vi "Write bombed.vi"(8 "error in (no error)":errorcluster, 10 "bombed":bool, 11 "BombedWall in":refnum<class "BombedWall.lvclass">) -> (0 "error out":errorcluster, 3 "BombedWall out":refnum<class "BombedWall.lvclass">)   [LabVIEW 2016, in "BombedWall.lvclass"]
uses:
  BombedWall.lvclass
  BombedWall.lvclass/BombedWall.ctl
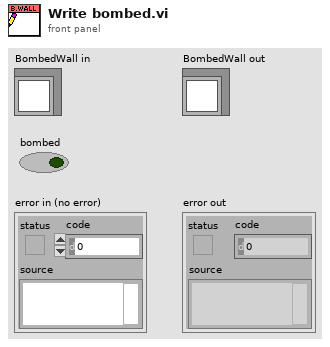
[diagram p1: front panel]
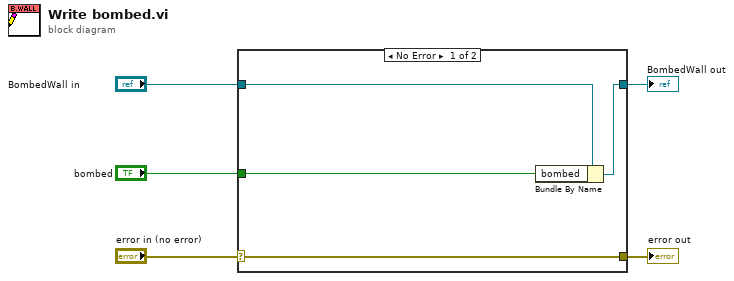
[diagram p0: block diagram]
diagram:
  n1 = case shown="No Error" "error in (no error)" {
    selector: "error in (no error)" -> [w9 w10]
    tunnel: [w9 w10] -> w4
    tunnel: [w7 w11] -> w2
    tunnel: "BombedWall in" -> [w8 w11]
    tunnel: "bombed" -> [w6 _]
    frame No Error {
      n2 = Bundle By Name(cluster=w8, "bombed"=w6) -> (w7:refnum<class "BombedWall.lvclass">)
    }
    frame Error {
    }
  }
  "error out" <- w4
  "BombedWall out" <- w2
